vi "Discrete Inverse CDF.vi"   [LabVIEW 2020, in "NI_Gmath.lvlib"]
doc: "Computes the discrete inverse cumulative distribution function (CDF), or the value <B>x</B> such that the probability that the random variate X, where X describes the selected distribution type, takes on a value less than or equal to it is <B>cdf(x)</B>. You must manually select the polymorphic instance to use."
uses:
  <vilib>/gmath/NI_Gmath.lvlib
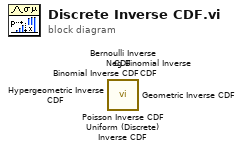
[diagram p0: block diagram]
diagram:
  n1 = call <vilib>:"Poisson Inverse CDF.vi"() -> ()  [unwired: 10 in, 2 out]
  n2 = call <vilib>:"Neg Binomial Inverse CDF.vi"() -> ()  [unwired: 10 in, 2 out]
  n3 = call <vilib>:"Hypergeometric Inverse CDF.vi"() -> ()  [unwired: 10 in, 2 out]
  n4 = call <vilib>:"Geometric Inverse CDF.vi"() -> ()  [unwired: 10 in, 2 out]
  n5 = call <vilib>:"Uniform (Discrete) Inverse CDF.vi"() -> ()  [unwired: 10 in, 2 out]
  n6 = call <vilib>:"Binomial Inverse CDF.vi"() -> ()  [unwired: 10 in, 2 out]
  n7 = call <vilib>:"Bernoulli Inverse CDF.vi"() -> ()  [unwired: 10 in, 2 out]
